vi "BIO_do_connect_accept_handshake_low_level.vi"(8 "error in (no error)":errorcluster, 11 "BIO in":refnum<class "BIO.lvclass">) -> (0 "error out":errorcluster, 2 "return type":i32, 3 "BIO out":refnum<class "BIO.lvclass">)   [LabVIEW 2013, in "SSL_Lib.lvlib" / "BIO.lvclass"]
uses:
  BIO.lvclass
  SSL-Lib/SSL-Lib.lvclass/SSL-Lib.ctl
  BIO.lvclass/BIO.ctl
  SSL-Lib/Read Crypto Library Path.vi
  Read Handle.vi
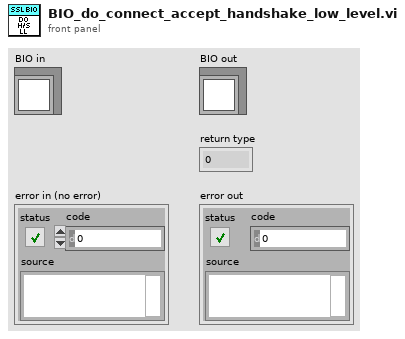
[diagram p1: front panel]
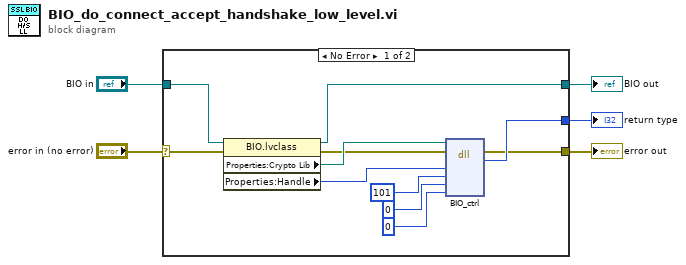
[diagram p0: block diagram]
diagram:
  n1 = case shown="No Error" "error in (no error)" {
    selector: "error in (no error)" -> [w6 w18]
    tunnel: [w16 _] -> w5
    tunnel: [w15 w18] -> w4
    tunnel: "BIO in" -> [w8 w17]
    tunnel: [w7 w17] -> w2
    frame No Error {
      n2 = property class="BIO.lvclass"(reference=w8, error in=w6) -> (reference out=w7:refnum<class "BIO.lvclass">, error out=w12:errorcluster, "Properties:Crypto Lib"=w13:path, "Properties:Handle"=w14:u64)
      n3 = dll-call lib="C:/Program Files (x86)/National Instruments/Shared/nissl/NIlibeay32.dll" fn="BIO_ctrl"(path in=w13, error in=w12, "BIO"=w14, "cmd"=101, "larg"=0, "parg"=0 ("larg")) -> (error out=w15:errorcluster, "return type"=w16:i32)  [unwired: 5 in, 1 out]
    }
    frame Error {
    }
  }
  "return type" <- w5
  "error out" <- w4
  "BIO out" <- w2
